vi "Parse Channel Name.vi"(1 "Channel Name":string) -> (0 "Channel":i32)   [LabVIEW 2017, in "XYStage.KIM101.lvclass"]
uses:
  XYStage.KIM101.lvclass
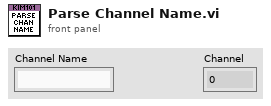
[diagram p1: front panel]
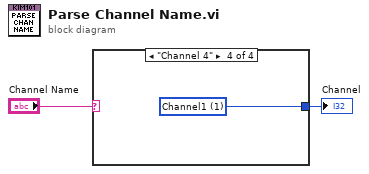
[diagram p0: block diagram]
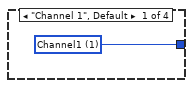
[diagram p2: hidden frame]
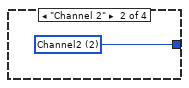
[diagram p3: hidden frame]
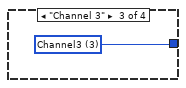
[diagram p4: hidden frame]
diagram:
  n1 = case shown="\"Channel 4\"" "Channel Name" {
    tunnel: [w3 w4 w5 w6] -> w1
    frame "Channel 1", Default {
      w3 = 1 items=["Channel1"=1, "Channel2"=2, "Channel3"=3, "Channel4"=4] ("channel")
    }
    frame "Channel 2" {
      w4 = 2 items=["Channel1"=1, "Channel2"=2, "Channel3"=3, "Channel4"=4] ("channel")
    }
    frame "Channel 3" {
      w5 = 3 items=["Channel1"=1, "Channel2"=2, "Channel3"=3, "Channel4"=4] ("channel")
    }
    frame "Channel 4" {
      w6 = 1 items=["Channel1"=1, "Channel2"=2, "Channel3"=3, "Channel4"=4] ("channel")
    }
  }
  "Channel" <- w1
